vi "Boiler System Open.vi"(8 "error in":errorcluster) -> (0 "error out":errorcluster, 1 "output cluster":T1, 2 "Notifiers":T3, 3 "Message Queues":T2, 5 "User Event - Stop":refnum<user-event>, 7 "Stop Event Registration Refnum":refnum<event-registration>)   [LabVIEW 2015]
uses:
  Notifiers/Notifiers.ctl
  Message Queue/All Message Queues.ctl
  Message Queue/Message Cluster.ctl
  controls/MHL Configuration.ctl
  User Event - Stop/User Event - Stop.lvlib
  Message Queue/Message Queue.lvlib
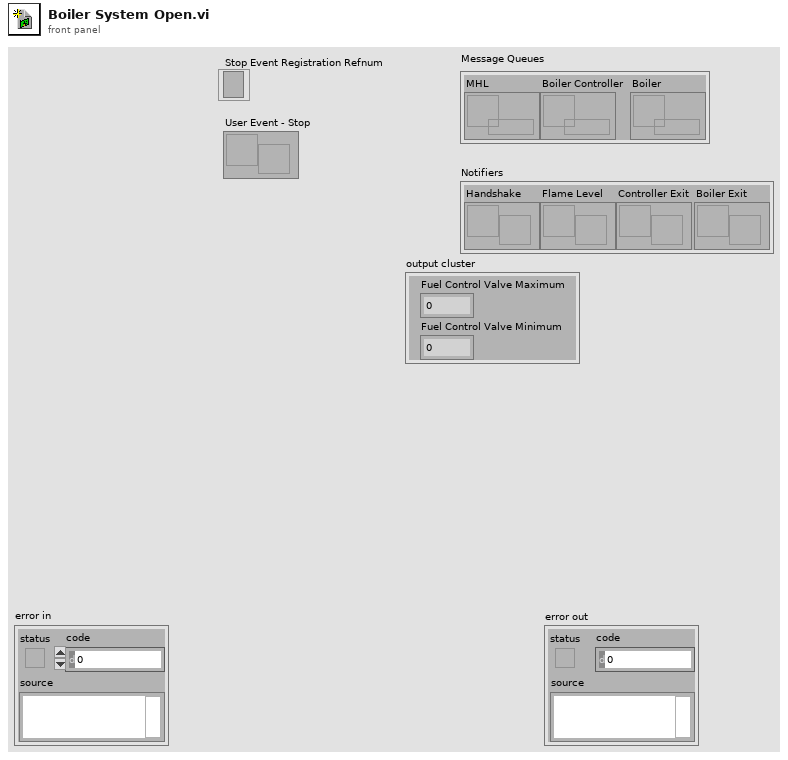
[diagram p1: front panel]
types:
  T1 = typedef "MHL Configuration.ctl" = cluster{"Fuel Control Valve Maximum":dbl, "Fuel Control Valve Minimum":dbl}
  T2 = typedef "Message Queue.lvlib/All Message Queues.ctl" = cluster{"MHL":refnum<queue>, "Boiler Controller":refnum<queue>, "Boiler":refnum<queue>}
  T3 = typedef "Notifiers.ctl" = cluster{"Handshake":refnum<notifier>, "Flame Level":refnum<notifier>, "Controller Exit":refnum<notifier>, "Boiler Exit":refnum<notifier>}
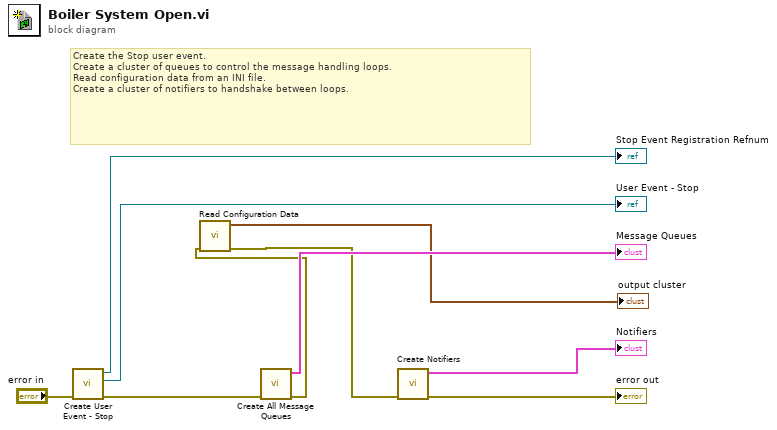
[diagram p0: block diagram]
diagram:
  # "Create the Stop user event.\nCreate a cluster of queues to control the message handling loops.\nRead configuration data from an INI file.\nCreate a cluster of notifiers to handshake between loops."
  n1 = call "Create User Event - Stop.vi"("error in (no error)"="error in") -> ("error out"=w10:errorcluster, "User Event - Stop"=→"User Event - Stop":refnum<user-event>, "Stop Event Registration Refnum"=→"Stop Event Registration Refnum":refnum<event-registration>)  [unwired: 8 in]
  n2 = call "Create All Message Queues.vi"("error in"=w10) -> ("error out"=w3:errorcluster, "Message Queues out"=→"Message Queues":T2)  [unwired: 9 in]
  n3 = call "Read Configuration Data.vi"("error in (no error)"=w3) -> ("error out"=w2:errorcluster, "output cluster"=→"output cluster":T1)  [unwired: 9 in]
  n4 = call "Create Notifiers.vi"("error in"=w2) -> ("error out"=→"error out":errorcluster, "Notifiers"=→"Notifiers":T3)  [unwired: 9 in]
